vi "Unlock.vi"(8 "error in (no error)":errorcluster, 11 "Timed Door in":refnum<class "Timed Door.lvclass">) -> (0 "error out":errorcluster, 3 "Timed Door out":refnum<class "Timed Door.lvclass">)   [LabVIEW 2018, in "Timed Door.lvclass"]
uses:
  Timed Door.lvclass
  Timer/Timer.lvclass
  Timed Door.lvclass/Timed Door.ctl
  Timer/Timer.lvclass/Timer.ctl
  Timer/Get Target Time Elapsed Event.vi
  Set Timer DVR.vi
  Set Target Time Elapsed Event.vi
  Set Alarm DVR.vi
  Door/Door.lvclass
  Alarm/Alarm.lvclass
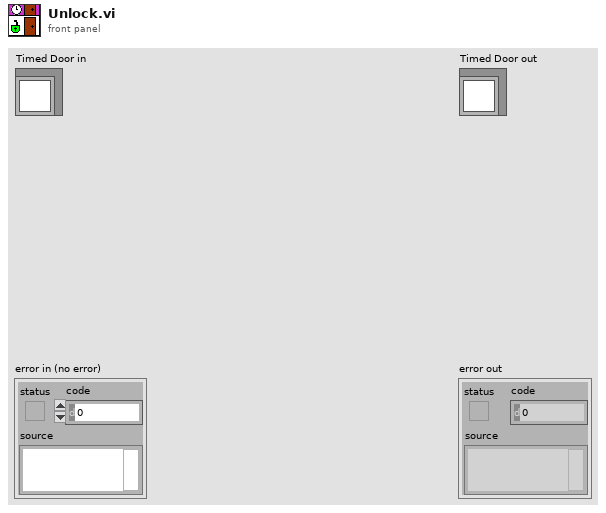
[diagram p1: front panel]
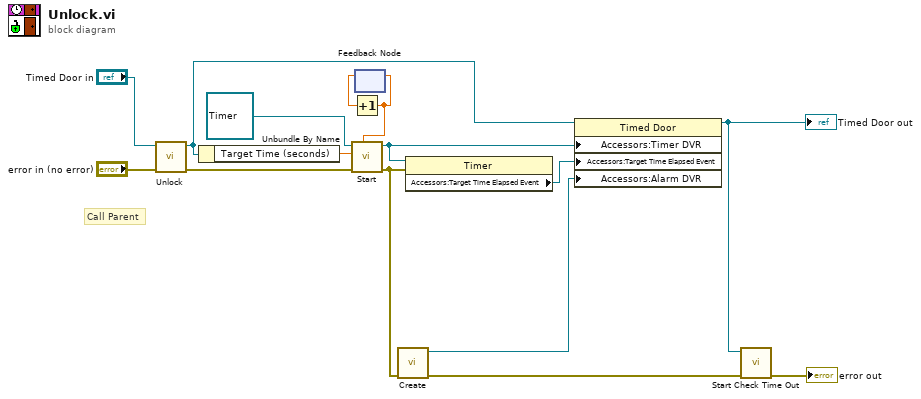
[diagram p0: block diagram]
diagram:
  # "Call Parent"
  n1 = call-parent "Unlock.vi"("error in (no error)"="error in (no error)", "Door in"="Timed Door in") -> ("error out"=w11:errorcluster, "Door out"=w9:refnum<class "Timed Door.lvclass">)  [unwired: 8 in]
  n2 = Unbundle By Name(w9) -> ("Target Time (seconds)"=w13:dbl)
  n3 = feedback #1() -> (w2:dbl)  [unwired: 1 in]
  n4 = Increment(x=w2) -> (x+1=w1:dbl)
  n5 = call-dynamic "Start.vi"("Timer ID"=w1, "error in (no error)"=w11, "Target Time (seconds)"=w13, "Timer in"=refnum<class "Timer.lvclass"> refnum) -> ("error out"=w5:errorcluster, "Timer DVR"=w4:refnum<data-value>)  [unwired: 6 in]
  n6 = feedback-in #1(w1) -> ()
  n7 = call "Create.vi"("error in (no error)"=w5) -> ("error out"=w6:errorcluster, "Alarm DVR"=w8:refnum<data-value>)  [unwired: 9 in]
  n8 = property class="Timer"(reference=w4, error in=w5) -> ("Accessors:Target Time Elapsed Event"=w3:refnum<user-event>)  [unwired: 2 out]
  n9 = property class="Timed Door"(reference=w9, "Accessors:Timer DVR"=w4, "Accessors:Target Time Elapsed Event"=w3, "Accessors:Alarm DVR"=w8) -> (reference out=w7:refnum<class "Timed Door.lvclass">)  [unwired: 1 in, 1 out]
  "Timed Door out" <- w7
  n10 = call "Start Check Time Out.vi"("error in (no error)"=w6, "Timed Door in"=w7) -> ("error out"=→"error out":errorcluster)  [unwired: 9 in]
